vi "Main.vi"() -> ()   [LabVIEW 2019]
uses:
  Image Acquisition Class/Camera.lvclass
panel:
  in  "Stop":bool
  out "Image":T1(plugin-control)
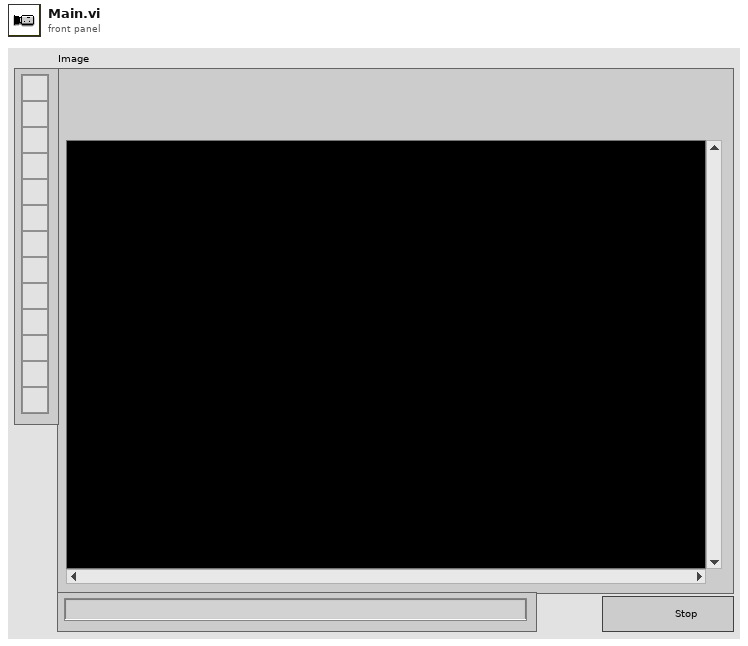
[diagram p1: front panel]
types:
  T1 = typedef "IMAQ Image.ctl" = refnum<image>
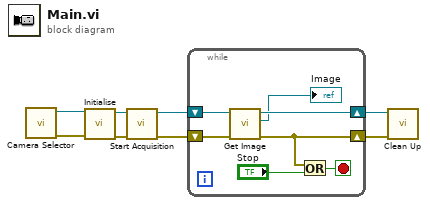
[diagram p0: block diagram]
diagram:
  n1 = call "Camera Selector.vi"() -> ("error out"=w1:errorcluster, "Image Acquisition out"=w2:refnum<class "Camera.lvclass">)  [unwired: 10 in]
  n2 = call-dynamic "Initialise.vi"("error in (no error)"=w1, "Image Acquisition in"=w2) -> ("error out"=w7:errorcluster, "Image Acquisition out"=w8:refnum<class "Camera.lvclass">)  [unwired: 8 in]
  n3 = call-dynamic "Start Acquisition.vi"("error in (no error)"=w7, "Image Acquisition in"=w8) -> ("error out"=w5:errorcluster, "Image Acquisition out"=w6:refnum<class "Camera.lvclass">)  [unwired: 8 in]
  n4 = while {
    shift-right: [w13] -> w4
    shift-left: w6 -> [w15]
    shift-right: [w11] -> w3
    shift-left: w5 -> [w14]
    stop <- w9 stop-if-true
    n5 = call-dynamic "Get Image.vi"("error in (no error)"=w14, "Image Acquisition in"=w15) -> ("error out"=w11:errorcluster, "Image Reference"=→"Image":T1, "Image Acquisition out"=w13:refnum<class "Camera.lvclass">)  [unwired: 7 in]
    n6 = Or(x=w11, y="Stop") -> (x .or. y?=w9:bool)
  }
  n7 = call-dynamic "Clean Up.vi"("error in (no error)"=w3, "Image Acquisition in"=w4) -> ()  [unwired: 8 in, 2 out]
